vi "SeedFeeder.vi"() -> ()   [LabVIEW 2018]
uses:
  <vilib>/Analysis/NI_AALPro.lvlib
panel:
  in  "DAQmx Device Name":tag="Current_PXI_1"
  in  "Channel":i32=2
  out "Arithmetic Mean":dbl(slide) scale=0.0..2000.0
  in  "milliseconds to wait":u32=250
  out "M (seed)":cluster{"X":dbl[], "Y":dbl[]}[](graph)
  out "dM/dt (seed)":cluster{"X":dbl[], "Y":dbl[]}(graph)
  in  "stop":bool
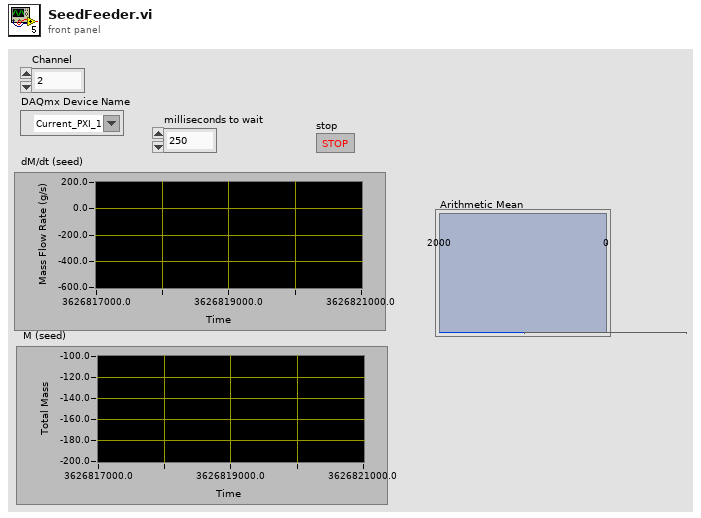
[diagram p1: front panel]
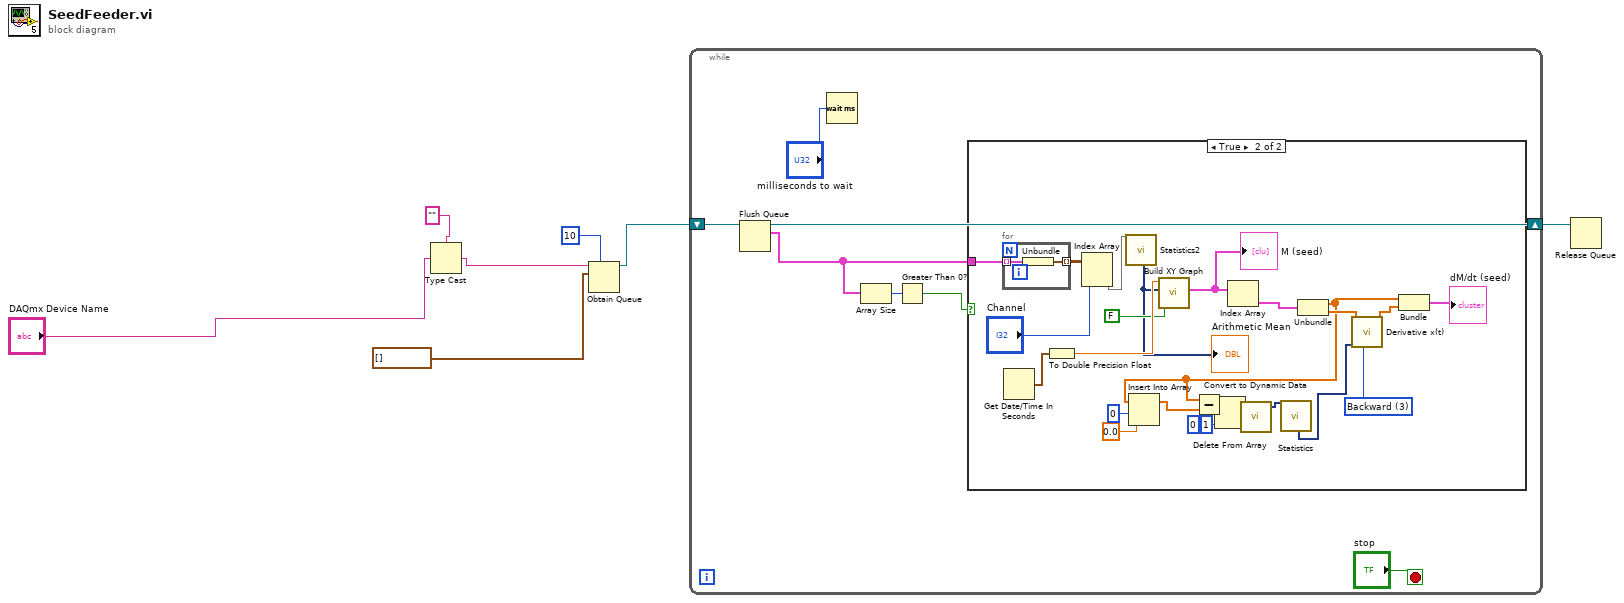
[diagram p0: block diagram]
diagram:
  n1 = Type Cast(type="", x="DAQmx Device Name") -> (*(type *) &x=w7:string)
  n2 = Obtain Queue(max queue size (-1, unlimited)=10, name (unnamed)=w7, element data type=waveform(dbl)[] [] ("data")) -> (queue out=w3:refnum<queue>)  [unwired: 2 in, 2 out]
  n3 = while {
    shift-right: [w13] -> w2
    shift-left: w3 -> [w14]
    stop <- "stop" stop-if-true
    n4 = Flush Queue(queue=w14) -> (queue out=w13:refnum<queue>, remaining elements=w10:cluster{"data":waveform(dbl)[]}[])  [unwired: 1 in, 1 out]
    n5 = Wait (ms)(milliseconds to wait="milliseconds to wait") -> ()  [unwired: 1 out]
    n6 = Array Size(array=w10) -> (size(s)=w9:i32)
    n7 = Greater Than 0?(x=w9) -> (x > 0?=w8:bool)
    n8 = case shown="True" w8 {
      tunnel: w10 -> [_ w38]
      frame False {
      }
      frame True {
        w31 = u16 3 items=["2nd Order Central", "4th Order Central", "Forward", "Backward"] ("method")
        n9 = for {
          tunnel: w38 -> [w40] mode=indexing
          tunnel: [w39] -> w37 mode=indexing
          n10 = Unbundle(w40) -> ("data"=w39:waveform(dbl)[])
        }
        n11 = Get Date/Time In Seconds() -> (seconds since 1Jan1904=w36:timestamp)
        n12 = To Double Precision Float(number=w36) -> (double precision float=w35:dbl)
        n13 = Index Array(array=w37, index (col)="Channel") -> (element=w22:waveform(dbl)[])  [unwired: 1 in]
        n14 = call "Statistics2"("Signals"=w22) -> ("Arithmetic Mean"=w21:dynamicdata)  [unwired: 25 in, 1 out]
        "Arithmetic Mean" <- w21
        n15 = call "Build XY Graph"("Reset"=FALSE, "Y Input"=w21, "X Input"=w35) -> ("XY Graph"=w20:cluster{"X":dbl[], "Y":dbl[]}[])  [unwired: 7 in, 1 out]
        "M (seed)" <- w20
        n16 = Index Array(array=w20) -> (element=w33:cluster{"X":dbl[], "Y":dbl[]})  [unwired: 1 in]
        n17 = Unbundle(w33) -> ("X"=w16:dbl[], "Y"=w32:dbl[])
        n18 = Insert Into Array(array=w16, index=0, new element=0.0 ("new element/subarray")) -> (w15:dbl[])
        n19 = Subtract(x=w16, y=w15) -> (x-y=w28:dbl[])
        n20 = Delete From Array(array=w28, length=1, index=0) -> (array with subset deleted=w19:dbl[])  [unwired: 1 out]
        n21 = call "Convert to Dynamic Data"("Array"=w19) -> ("Dynamic Data Type"=w27:dynamicdata)  [unwired: 3 in]
        n22 = call "Statistics"("Signals"=w27) -> ("Arithmetic Mean"=w26:dynamicdata)  [unwired: 25 in, 1 out]
        n23 = call <vilib>:"Derivative x(t).vi"("method"=w31, "dt"=w26, "X"=w32) -> ("dX/dt"=w30:dbl[])  [unwired: 7 in, 1 out]
        n24 = Bundle("X"=w16, "dX/dt"=w30) -> (→"dM/dt (seed)":cluster{"X":dbl[], "dX/dt":dbl[]})  [unwired: 1 in]
      }
    }
  }
  n25 = Release Queue(queue=w2) -> ()  [unwired: 2 in, 3 out]
